vi "Writetofile_NeverOverwrite.vi"(9 "appended array":dbl[](array[numeric]), 11 "FilePathOut":path) -> ()   [LabVIEW 2014]
uses:
  <vilib>/Utility/file.llb/Write To Spreadsheet File (DBL).vi
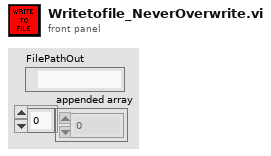
[diagram p1: front panel]
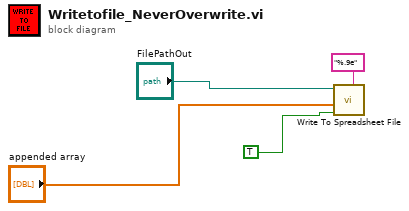
[diagram p0: block diagram]
diagram:
  n1 = call-poly <vilib>:"Write To Spreadsheet File.vi"("format (%.3f)"="%.9e", "append to file? (new file:F)"=TRUE, "1D data"="appended array", "file path (dialog if empty)"="FilePathOut") -> ()  [unwired: 4 in, 1 out]
